vi "Configure.vi"(8 "error in (no error)":errorcluster, 11 "GRMActor in":refnum<class "Displayer.lvclass">) -> (0 "error out":errorcluster, 3 "GRMActor out":refnum<class "Displayer.lvclass">)   [LabVIEW 2020, in "Displayer.lvlib" / "Displayer.lvclass"]
uses:
  Displayer.lvclass
  Model/Hardware Abstraction Layer/Component/GenericActor/GenericActor/GenericActor.lvclass
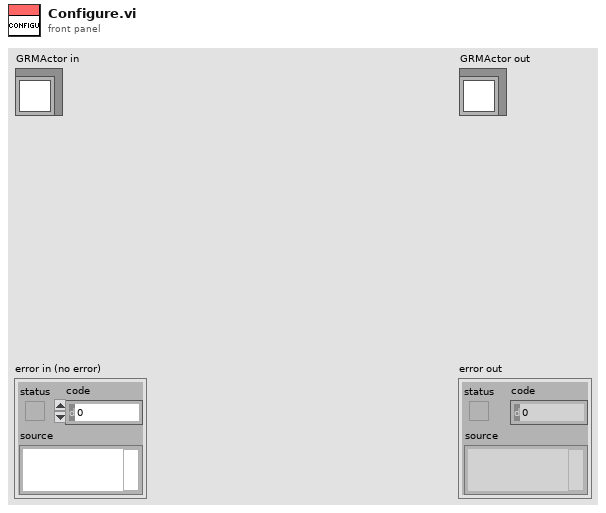
[diagram p1: front panel]
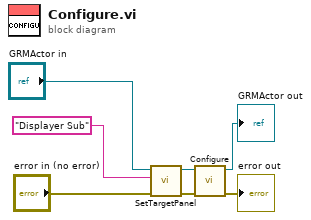
[diagram p0: block diagram]
diagram:
  n1 = call-dynamic "SetTargetPanel.vi"("error in (no error)"="error in (no error)", "TargetPanel"="Displayer Sub", "GRMActor in"="GRMActor in") -> ("error out"=w4:errorcluster, "GRMActor out"=w2:refnum<class "Displayer.lvclass">)  [unwired: 7 in]
  n2 = call-parent "Configure.vi"("error in (no error)"=w4, "GRMActor in"=w2) -> ("error out"=→"error out":errorcluster, "GRMActor out"=→"GRMActor out":refnum<class "Displayer.lvclass">)  [unwired: 8 in]
